vi "SVL Integration (peaks) (1 Ch).vi"(0 "peaks":cluster{"frequency [Hz]":dbl, "value":dbl}[](array[cluster]) {"value" format="%.2f"; "frequency [Hz]" format="%.2f"}, 1 "integration type":T7(ring)=enum."double integration", 4 "spectrum info in":T1={"channel name"="", "description"="", "x-axis units"=0, "spectral info"={"spectrum type"=enum."Power [Magnitude^2]", "linear/dB"=enum."linear", "window"=0, "window size"=0, "FFT size"=0}, "engineering units"=0, "custom label"="", "dB reference [EU]"=0.0, "peak units"=enum."rms", "weighting filter"=0, "spectral density?"=FALSE, "unit label"="", "spectrum skewed?"=FALSE, "complimentary spectrum units"=enum."none"} {"x-axis units" items=["Time (s)"=0, "Frequency-CB (Hz)"=1, "Frequency-CPB (Hz)"=1248, "Frequency-Arbitrary (Hz)"=2357, "Quefrency (s)"=2, "Revolutions (rev)"=3, "Order"=4, "Speed (RPM)"=11, "Speed (rad/s)"=21, "Index"=65535]; "weighting filter" items=["Linear", "A-weighting", "B-weighting", "C-weighting", "ITU-R 468-4", "Dolby", "CCITT", "C-message", "Wb", "Wc", "Wd", "We", "Wf", "Wh", "Wj", "Wk", "Wm", "AES17 20 kHz lowpass", "AES17 40 kHz lowpass", "AES17 20 kHz highpass", "AES17 40 kHz highpass"]; "dB reference [EU]" format="%.2f"; "engineering units" items=["custom..."=0, "V"=1, "A"=21, "C"=30, "pC"=31, "s"=32, "-"=29, "Pa"=2, "N"=20, "g"=3, "m/s^2"=4, "m/s"=5, "m"=6, "mm/s"=12, "mm"=13, "micron/s"=14, "micron"=15, "in/s^2"=7, "in/s"=8, "in"=9, "mil/s"=10, "mil"=11, "rad/s^2"=16, "rad/s"=17, "rad"=18, "deg/s^2"=26, "deg/s"=27, "deg"=28, "RPM"=22, "cycle/s^2"=23, "Hz"=24, "cycle"=25, "strain"=19]; "spectral info"."window" items=["None "=0, "Hanning"=1, "Hamming"=2, "Blackman-Harris"=3, "Exact Blackman"=4, "Blackman"=5, "Flat Top"=6, "4 Term B-Harris "=7, "7 Term B-Harris"=8, "Low Sidelobe"=9, "Force - Exponential"=10, "Gaussian"=62]}, 5 "error in (no error)":errorcluster, 6 "length units":i32(ring) items=["no change"=-1, "m"=0, "mm"=2, "microns"=3, "in"=1, "mils"=5]) -> (14 "integrated peaks":cluster{"frequency [Hz]":dbl, "value":dbl}[](array[cluster]) {"value" format="%.2f"; "frequency [Hz]" format="%.2f"}, 15 "unit label":string, 18 "spectrum info out":T1={"channel name"="", "description"="", "x-axis units"=0, "spectral info"={"spectrum type"=enum."Power [Magnitude^2]", "linear/dB"=enum."linear", "window"=0, "window size"=0, "FFT size"=0}, "engineering units"=0, "custom label"="", "dB reference [EU]"=0.0, "peak units"=enum."rms", "weighting filter"=0, "spectral density?"=FALSE, "unit label"="", "spectrum skewed?"=FALSE, "complimentary spectrum units"=enum."none"} {"x-axis units" items=["Time (s)"=0, "Frequency-CB (Hz)"=1, "Frequency-CPB (Hz)"=1248, "Frequency-Arbitrary (Hz)"=2357, "Quefrency (s)"=2, "Revolutions (rev)"=3, "Order"=4, "Speed (RPM)"=11, "Speed (rad/s)"=21, "Index"=65535]; "weighting filter" items=["Linear", "A-weighting", "B-weighting", "C-weighting", "ITU-R 468-4", "Dolby", "CCITT", "C-message", "Wb", "Wc", "Wd", "We", "Wf", "Wh", "Wj", "Wk", "Wm", "AES17 20 kHz lowpass", "AES17 40 kHz lowpass", "AES17 20 kHz highpass", "AES17 40 kHz highpass"]; "dB reference [EU]" format="%.2f"; "engineering units" items=["custom..."=0, "V"=1, "A"=21, "C"=30, "pC"=31, "s"=32, "-"=29, "Pa"=2, "N"=20, "g"=3, "m/s^2"=4, "m/s"=5, "m"=6, "mm/s"=12, "mm"=13, "micron/s"=14, "micron"=15, "in/s^2"=7, "in/s"=8, "in"=9, "mil/s"=10, "mil"=11, "rad/s^2"=16, "rad/s"=17, "rad"=18, "deg/s^2"=26, "deg/s"=27, "deg"=28, "RPM"=22, "cycle/s^2"=23, "Hz"=24, "cycle"=25, "strain"=19]; "spectral info"."window" items=["None "=0, "Hanning"=1, "Hamming"=2, "Blackman-Harris"=3, "Exact Blackman"=4, "Blackman"=5, "Flat Top"=6, "4 Term B-Harris "=7, "7 Term B-Harris"=8, "Low Sidelobe"=9, "Force - Exponential"=10, "Gaussian"=62]}, 19 "error out":errorcluster)   [LabVIEW 2017, in "SoundVib_Integration.lvlib"]
doc: "Converts acceleration to velocity or displacement using a frequency spectrum as the input. Wire data to the <B>spectrum</B> input to determine the polymorphic instance to use or manually select the instance."
uses:
  <vilib>/addons/Sound and Vibration/svt_Integration/SoundVib_Integration.lvlib
  <vilib>/addons/_NISVFA/_Shared subVIs/Controls/svc_Spectrum Info.ctl
  <vilib>/addons/_NISVFA/_Shared subVIs/Controls/svc_X-Axis Units.ctl
  <vilib>/addons/_NISVFA/_Shared subVIs/Controls/svc_Spectrum Type.ctl
  <vilib>/addons/_NISVFA/_Shared subVIs/Controls/svc_Engineering Units Text Ring.ctl
  <vilib>/addons/_NISVFA/_Shared subVIs/Controls/svc_Weighting Filter Text Ring.ctl
  <vilib>/addons/_NISVFA/_Shared subVIs/Controls/svc_Complimentary Spectrum Units.ctl
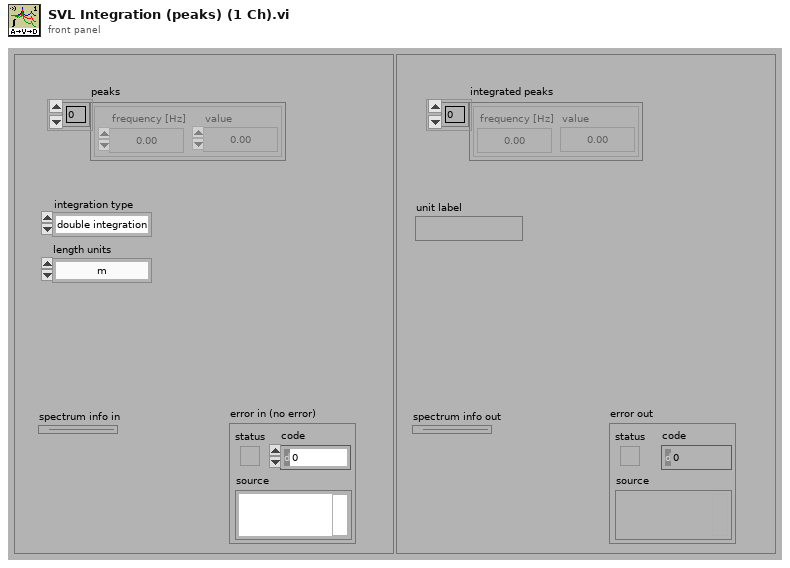
[diagram p1: front panel]
types:
  T1 = typedef "svc_Spectrum Info.ctl" = cluster{"channel name":string, "description":string, "x-axis units":T2, "spectral info":cluster{"spectrum type":T3, "linear/dB":enum16{"linear", "dB"}, "window":u16, "window size":i32, "FFT size":i32}, "engineering units":T4, "custom label":string, "dB reference [EU]":dbl, "peak units":enum16{"rms", "peak", "peak-peak"}, "weighting filter":T5, "spectral density?":bool, "unit label":string, "spectrum skewed?":bool, "complimentary spectrum units":T6}
  T2 = typedef "svc_X-Axis Units.ctl" = u16
  T3 = typedef "svc_Spectrum Type.ctl" = enum16{"FFT Spectrum [complex]", "Amplitude [Magnitude]", "Power [Magnitude^2]", "Cross Spectrum [complex]", "Frequency Response [Complex]"}
  T4 = typedef "svc_Engineering Units Text Ring.ctl" = u16
  T5 = typedef "svc_Weighting Filter Text Ring.ctl" = u16
  T6 = typedef "svc_Complimentary Spectrum Units.ctl" = enum16{"none", "radians", "degrees", "cycles", "imaginary"}
  T7 = enum16{"single integration", "double integration"}
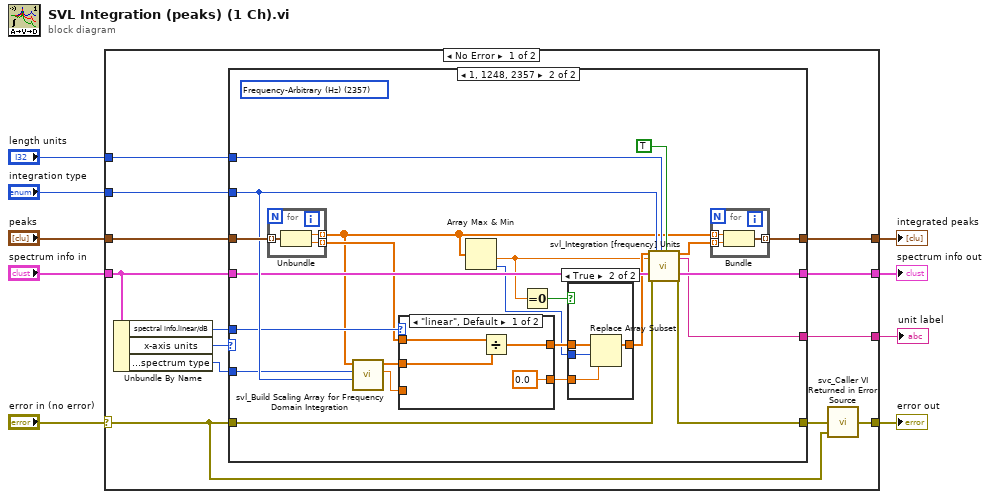
[diagram p0: block diagram]
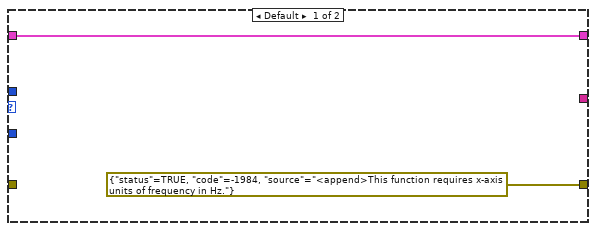
[diagram p2: hidden frame]
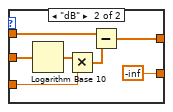
[diagram p4: hidden frame]
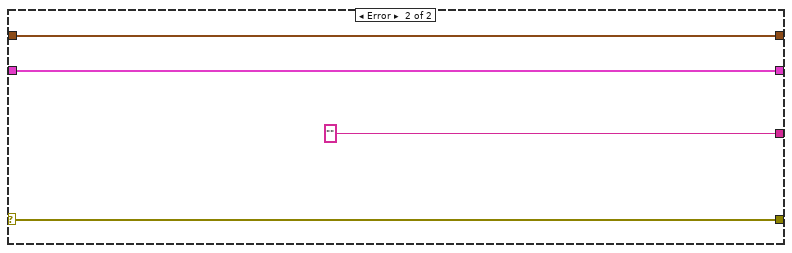
[diagram p5: hidden frame]
diagram:
  n1 = case shown="No Error" "error in (no error)" {
    selector: "error in (no error)" -> [w11 w72]
    tunnel: [w22 w73] -> w9
    tunnel: "peaks" -> [w21 w73]
    tunnel: "integration type" -> [w20 _]
    tunnel: "spectrum info in" -> [w17 w71]
    tunnel: [w12 w72] -> w4
    tunnel: [w16 w71] -> w3
    tunnel: "length units" -> [w15 _]
    tunnel: [w14 "" ("unit label")] -> w1
    frame No Error {
      n2 = Unbundle By Name(w17) -> ("spectral info.linear/dB"=w19:enum16{"linear", "dB"}, "x-axis units"=w10:T2, "spectral info.spectrum type"=w13:T3)
      n3 = case shown="1, 1248, 2357" w10 {
        tunnel: [_ w47] -> w22
        tunnel: w21 -> [_ w46]
        tunnel: w20 -> [_ w45]
        tunnel: w19 -> [_ w44]
        tunnel: [errorcluster {"status"=TRUE, "code"=-1984, "source"="<append>This function requires x-axis units of frequency in Hz."} ("error out") w43] -> w18
        tunnel: w17 -> [w24 w42]
        tunnel: [w24 w41] -> w16
        tunnel: w15 -> [_ w40]
        tunnel: [_ w39] -> w14
        tunnel: w13 -> [_ w38]
        tunnel: w11 -> [_ w37]
        frame Default {
        }
        frame 1, 1248, 2357 {
          (unwired) T2 2357 items=["Time (s)"=0, "Frequency-CB (Hz)"=1, "Frequency-CPB (Hz)"=1248, "Frequency-Arbitrary (Hz)"=2357, "Quefrency (s)"=2, "Revolutions (rev)"=3, "Order"=4, "Speed (RPM)"=11, "Speed (rad/s)"=21, "Critical Band"=31, "Critical Band Rate (Bark)"=32, "None"=98, "Index"=65535] ("x-axis units")
          n4 = for {
            tunnel: w46 -> [w53] mode=indexing
            tunnel: [w52] -> w26 mode=indexing
            tunnel: [w51] -> w28 mode=indexing
            n5 = Unbundle(w53) -> ("frequency [Hz]"=w52:dbl, "value"=w51:dbl)
          }
          n6 = call <vilib>:"svl_Build Scaling Array for Frequency Domain Integration.vi"("integration type"=w45, "spectrum type"=w38, "frequency array [Hz]"=w26) -> ("dB multiplier"=w32:dbl, "scaling array"=w31:dbl[])  [unwired: 7 in]
          n7 = case shown="\"linear\", Default" w44 {
            tunnel: w28 -> [w62 w66]
            tunnel: [w60 w64] -> w36
            tunnel: w31 -> [w61 w69]
            tunnel: w32 -> [_ w67]
            tunnel: [0.0 ("New Element/Subarray") -inf] -> w34
            frame "linear", Default {
              n8 = Divide(x=w62, y=w61) -> (x/y=w60:dbl[])
            }
            frame "dB" {
              n9 = Logarithm Base 10(1:w69) -> (0:w68:dbl[])
              n10 = Multiply(x=w68, y=w67) -> (x*y=w65:dbl[])
              n11 = Subtract(x=w66, y=w65) -> (x-y=w64:dbl[])
            }
          }
          n12 = Array Max & Min(array=w26) -> (min value=w29:dbl, min index (indices)=w27:i32)  [unwired: 2 out]
          n13 = Equal To 0?(x=w29) -> (x = 0?=w35:bool)
          n14 = case shown="True" w35 {
            tunnel: w36 -> [w54 w58]
            tunnel: [w54 w57] -> w30
            tunnel: w34 -> [_ w56]
            tunnel: w27 -> [_ w55]
            frame False {
            }
            frame True {
              n15 = Replace Array Subset(array=w58, new element=w56, index=w55) -> (w57:dbl[])
            }
          }
          n16 = call <vilib>:"svl_Integration [frequency] Units.vi"("spectrum"=w30, "f0"=w29, "spectrum info in"=w42, "error in"=w37, "integration type"=w45, "desired base units for length"=w40, "automatically convert peak units"=TRUE ("convert displacement to peak units")) -> ("spectrum"=w25:dbl[], "unit label"=w39:string, "spectrum info out"=w41:T1, "error out"=w43:errorcluster)  [unwired: 9 in]
          n17 = for {
            tunnel: w26 -> [w50] mode=indexing
            tunnel: w25 -> [w49] mode=indexing
            tunnel: [w48] -> w47 mode=indexing
            n18 = Bundle("frequency [Hz]"=w50, w49) -> (w48:cluster{"frequency [Hz]":dbl, dbl})  [unwired: 1 in]
          }
        }
      }
      n19 = call <vilib>:"svc_Caller VI Returned in Error Source.vi"("warning input to caller"=w11, "error in (no error)"=w18) -> ("error out"=w12:errorcluster)  [unwired: 3 in]
    }
    frame Error {
    }
  }
  "integrated peaks" <- w9
  "error out" <- w4
  "spectrum info out" <- w3
  "unit label" <- w1
